vi "test TCX read (installed 71).vi"() -> ()   [LabVIEW 2011] (continued)
50</Watts></TPX></Extensions></Trackpoint><Trackpoint><Time>2008-03-03T13:52:56Z</Time><Position><LatitudeDegrees>35.876040</LatitudeDegrees><LongitudeDegrees>-78.942872</LongitudeDegrees></Position><AltitudeMeters>71.755</AltitudeMeters><DistanceMeters>2722.578</DistanceMeters><Cadence>80</Cadence><Extensions><TPX xmlns=\"http://www.garmin.com/xmlschemas/ActivityExtension/v2\"><Watts>198</Watts></TPX></Extensions></Trackpoint><Trackpoint><Time>2008-03-03T13:52:57Z</Time><Position><LatitudeDegrees>35.876036</LatitudeDegrees><LongitudeDegrees>-78.942746</LongitudeDegrees></Position><AltitudeMeters>71.755</AltitudeMeters><DistanceMeters>2733.887</DistanceMeters><Cadence>79</Cadence><Extensions><TPX xmlns=\"http://www.garmin.com/xmlschemas/ActivityExtension/v2\"><Watts>206</Watts></TPX></Extensions></Trackpoint><Trackpoint><Time>2008-03-03T13:52:58Z</Time><Position><LatitudeDegrees>35.876038</LatitudeDegrees><LongitudeDegrees>-78.942624</LongitudeDegrees></Position><AltitudeMeters>71.755</AltitudeMeters><DistanceMeters>2744.982</DistanceMeters><Cadence>76</Cadence><Extensions><TPX xmlns=\"http://www.garmin.com/xmlschemas/ActivityExtension/v2\"><Watts>226</Watts></TPX></Extensions></Trackpoint><Trackpoint><Time>2008-03-03T13:52:59Z</Time><Position><LatitudeDegrees>35.876041</LatitudeDegrees><LongitudeDegrees>-78.942503</LongitudeDegrees></Position><AltitudeMeters>72.236</AltitudeMeters><DistanceMeters>2755.792</DistanceMeters><Cadence>76</Cadence><Extensions><TPX xmlns=\"http://www.garmin.com/xmlschemas/ActivityExtension/v2\"><Watts>230</Watts></TPX></Extensions></Trackpoint><Trackpoint><Time>2008-03-03T13:53:00Z</Time><Position><LatitudeDegrees>35.876046</LatitudeDegrees><LongitudeDegrees>-78.942386</LongitudeDegrees></Position><AltitudeMeters>71.755</AltitudeMeters><DistanceMeters>2766.434</DistanceMeters><Cadence>76</Cadence><Extensions><TPX xmlns=\"http://www.garmin.com/xmlschemas/ActivityExtension/v2\"><Watts>228</Watts></TPX></Extensions></Trackpoint><Trackpoint><Time>2008-03-03T13:53:01Z</Time><Position><LatitudeDegrees>35.876052</LatitudeDegrees><LongitudeDegrees>-78.942271</LongitudeDegrees></Position><AltitudeMeters>72.236</AltitudeMeters><DistanceMeters>2776.748</DistanceMeters><Cadence>73</Cadence><Extensions><TPX xmlns=\"http://www.garmin.com/xmlschemas/ActivityExtension/v2\"><Watts>231</Watts></TPX></Extensions></Trackpoint><Trackpoint><Time>2008-03-03T13:53:02Z</Time><Position><LatitudeDegrees>35.876061</LatitudeDegrees><LongitudeDegrees>-78.942160</LongitudeDegrees></Position><AltitudeMeters>72.236</AltitudeMeters><DistanceMeters>2786.833</DistanceMeters><Cadence>71</Cadence><Extensions><TPX xmlns=\"http://www.garmin.com/xmlschemas/ActivityExtension/v2\"><Watts>227</Watts></TPX></Extensions></Trackpoint><Trackpoint><Time>2008-03-03T13:53:03Z</Time><Position><LatitudeDegrees>35.876074</LatitudeDegrees><LongitudeDegrees>-78.942052</LongitudeDegrees></Position><AltitudeMeters>72.236</AltitudeMeters><DistanceMeters>2796.726</DistanceMeters><Cadence>68</Cadence><Extensions><TPX xmlns=\"http://www.garmin.com/xmlschemas/ActivityExtension/v2\"><Watts>222</Watts></TPX></Extensions></Trackpoint><Trackpoint><Time>2008-03-03T13:53:04Z</Time><Position><LatitudeDegrees>35.876089</LatitudeDegrees><LongitudeDegrees>-78.941947</LongitudeDegrees></Position><AltitudeMeters>72.717</AltitudeMeters><DistanceMeters>2806.305</DistanceMeters><Cadence>68</Cadence><Extensions><TPX xmlns=\"http://www.garmin.com/xmlschemas/ActivityExtension/v2\"><Watts>231</Watts></TPX></Extensions></Trackpoint><Trackpoint><Time>2008-03-03T13:53:05Z</Time><Position><LatitudeDegrees>35.876106</LatitudeDegrees><LongitudeDegrees>-78.941844</LongitudeDegrees></Position><AltitudeMeters>72.717</AltitudeMeters><DistanceMeters>2815.787</DistanceMeters><Cadence>68</Cadence><Extensions><TPX xmlns=\"http://www.garmin.com/xmlschemas/ActivityExtension/v2\"><Watts>230</Watts></TPX></Extensions></Trackpoint><Trackpoint><Time>2008-03-03T13:53:06Z</Time><Position><LatitudeDegrees>35.876126</LatitudeDegrees><LongitudeDegrees>-78.941745</LongitudeDegrees></Position><AltitudeMeters>72.717</AltitudeMeters><DistanceMeters>2824.935</DistanceMeters><Cadence>65</Cadence><Extensions><TPX xmlns=\"http://www.garmin.com/xmlschemas/ActivityExtension/v2\"><Watts>244</Watts></TPX></Extensions></Trackpoint><Trackpoint><Time>2008-03-03T13:53:07Z</Time><Position><LatitudeDegrees>35.876144</LatitudeDegrees><LongitudeDegrees>-78.941647</LongitudeDegrees></Position><AltitudeMeters>73.198</AltitudeMeters><DistanceMeters>2834.040</DistanceMeters><Cadence>63</Cadence><Extensions><TPX xmlns=\"http://www.garmin.com/xmlschemas/ActivityExtension/v2\"><Watts>230</Watts></TPX></Extensions></Trackpoint><Trackpoint><Time>2008-03-03T13:53:08Z</Time><Position><LatitudeDegrees>35.876160</LatitudeDegrees><LongitudeDegrees>-78.941550</LongitudeDegrees></Position><AltitudeMeters>73.198</AltitudeMeters><DistanceMeters>2842.936</DistanceMeters><Cadence>62</Cadence><Extensions><TPX xmlns=\"http://www.garmin.com/xmlschemas/ActivityExtension/v2\"><Watts>222</Watts></TPX></Extensions></Trackpoint><Trackpoint><Time>2008-03-03T13:53:09Z</Time><Position><LatitudeDegrees>35.876180</LatitudeDegrees><LongitudeDegrees>-78.941457</LongitudeDegrees></Position><AltitudeMeters>73.678</AltitudeMeters><DistanceMeters>2851.633</DistanceMeters><Cadence>62</Cadence><Extensions><TPX xmlns=\"http://www.garmin.com/xmlschemas/ActivityExtension/v2\"><Watts>213</Watts></TPX></Extensions></Trackpoint><Trackpoint><Time>2008-03-03T13:53:10Z</Time><Position><LatitudeDegrees>35.876199</LatitudeDegrees><LongitudeDegrees>-78.941364</LongitudeDegrees></Position><AltitudeMeters>73.678</AltitudeMeters><DistanceMeters>2860.265</DistanceMeters><Cadence>66</Cadence><Extensions><TPX xmlns=\"http://www.garmin.com/xmlschemas/ActivityExtension/v2\"><Watts>203</Watts></TPX></Extensions></Trackpoint><Trackpoint><Time>2008-03-03T13:53:11Z</Time><Position><LatitudeDegrees>35.876216</LatitudeDegrees><LongitudeDegrees>-78.941272</LongitudeDegrees></Position><AltitudeMeters>73.678</AltitudeMeters><DistanceMeters>2868.794</DistanceMeters><Cadence>68</Cadence><Extensions><TPX xmlns=\"http://www.garmin.com/xmlschemas/ActivityExtension/v2\"><Watts>194</Watts></TPX></Extensions></Trackpoint><Trackpoint><Time>2008-03-03T13:53:12Z</Time><Position><LatitudeDegrees>35.876234</LatitudeDegrees><LongitudeDegrees>-78.941181</LongitudeDegrees></Position><AltitudeMeters>74.159</AltitudeMeters><DistanceMeters>2877.271</DistanceMeters><Cadence>69</Cadence><Extensions><TPX xmlns=\"http://www.garmin.com/xmlschemas/ActivityExtension/v2\"><Watts>188</Watts></TPX></Extensions></Trackpoint><Trackpoint><Time>2008-03-03T13:53:13Z</Time><Position><LatitudeDegrees>35.876255</LatitudeDegrees><LongitudeDegrees>-78.941091</LongitudeDegrees></Position><AltitudeMeters>73.198</AltitudeMeters><DistanceMeters>2885.719</DistanceMeters><Cadence>77</Cadence><Extensions><TPX xmlns=\"http://www.garmin.com/xmlschemas/ActivityExtension/v2\"><Watts>184</Watts></TPX></Extensions></Trackpoint><Trackpoint><Time>2008-03-03T13:53:14Z</Time><Position><LatitudeDegrees>35.876274</LatitudeDegrees><LongitudeDegrees>-78.941001</LongitudeDegrees></Position><AltitudeMeters>73.678</AltitudeMeters><DistanceMeters>2894.048</DistanceMeters><Cadence>77</Cadence><Extensions><TPX xmlns=\"http://www.garmin.com/xmlschemas/ActivityExtension/v2\"><Watts>183</Watts></TPX></Extensions></Trackpoint><Trackpoint><Time>2008-03-03T13:53:15Z</Time><Position><LatitudeDegrees>35.876290</LatitudeDegrees><LongitudeDegrees>-78.940913</LongitudeDegrees></Position><AltitudeMeters>74.159</AltitudeMeters><DistanceMeters>2902.261</DistanceMeters><Cadence>76</Cadence><Extensions><TPX xmlns=\"http://www.garmin.com/xmlschemas/ActivityExtension/v2\"><Watts>198</Watts></TPX></Extensions></Trackpoint><Trackpoint><Time>2008-03-03T13:53:16Z</Time><Position><LatitudeDegrees>35.876307</LatitudeDegrees><LongitudeDegrees>-78.940824</LongitudeDegrees></Position><AltitudeMeters>73.678</AltitudeMeters><DistanceMeters>2910.497</DistanceMeters><Cadence>76</Cadence><Extensions><TPX xmlns=\"http://www.garmin.com/xmlschemas/ActivityExtension/v2\"><Watts>206</Watts></TPX></Extensions></Trackpoint><Trackpoint><Time>2008-03-03T13:53:17Z</Time><Position><LatitudeDegrees>35.876319</LatitudeDegrees><LongitudeDegrees>-78.940734</LongitudeDegrees></Position><AltitudeMeters>74.159</AltitudeMeters><DistanceMeters>2918.685</DistanceMeters><Cadence>76</Cadence><Extensions><TPX xmlns=\"http://www.garmin.com/xmlschemas/ActivityExtension/v2\"><Watts>206</Watts></TPX></Extensions></Trackpoint><Trackpoint><Time>2008-03-03T13:53:18Z</Time><Position><LatitudeDegrees>35.876326</LatitudeDegrees><LongitudeDegrees>-78.940644</LongitudeDegrees></Position><AltitudeMeters>74.159</AltitudeMeters><DistanceMeters>2926.918</DistanceMeters><Cadence>76</Cadence><Extensions><TPX xmlns=\"http://www.garmin.com/xmlschemas/ActivityExtension/v2\"><Watts>198</Watts></TPX></Extensions></Trackpoint><Trackpoint><Time>2008-03-03T13:53:19Z</Time><Position><LatitudeDegrees>35.876330</LatitudeDegrees><LongitudeDegrees>-78.940552</LongitudeDegrees></Position><AltitudeMeters>73.678</AltitudeMeters><DistanceMeters>2935.164</DistanceMeters><Cadence>77</Cadence><Extensions><TPX xmlns=\"http://www.garmin.com/xmlschemas/ActivityExtension/v2\"><Watts>178</Watts></TPX></Extensions></Trackpoint><Trackpoint><Time>2008-03-03T13:53:20Z</Time><Position><LatitudeDegrees>35.876336</LatitudeDegrees><LongitudeDegrees>-78.940461</LongitudeDegrees></Position><AltitudeMeters>73.678</AltitudeMeters><DistanceMeters>2943.486</DistanceMeters><Cadence>77</Cadence><Extensions><TPX xmlns=\"http://www.garmin.com/xmlschemas/ActivityExtension/v2\"><Watts>165</Watts></TPX></Extensions></Trackpoint><Trackpoint><Time>2008-03-03T13:53:21Z</Time><Position><LatitudeDegrees>35.876341</LatitudeDegrees><LongitudeDegrees>-78.940369</LongitudeDegrees></Position><AltitudeMeters>74.640</AltitudeMeters><DistanceMeters>2951.737</DistanceMeters><Cadence>78</Cadence><Extensions><TPX xmlns=\"http://www.garmin.com/xmlschemas/ActivityExtension/v2\"><Watts>167</Watts></TPX></Extensions></Trackpoint><Trackpoint><Time>2008-03-03T13:53:22Z</Time><Position><LatitudeDegrees>35.876344</LatitudeDegrees><LongitudeDegrees>-78.940279</LongitudeDegrees></Position><AltitudeMeters>74.159</AltitudeMeters><DistanceMeters>2959.913</DistanceMeters><Cadence>77</Cadence><Extensions><TPX xmlns=\"http://www.garmin.com/xmlschemas/ActivityExtension/v2\"><Watts>184</Watts></TPX></Extensions></Trackpoint><Trackpoint><Time>2008-03-03T13:53:23Z</Time><Position><LatitudeDegrees>35.876339</LatitudeDegrees><LongitudeDegrees>-78.940189</LongitudeDegrees></Position><AltitudeMeters>74.159</AltitudeMeters><DistanceMeters>2968.036</DistanceMeters><Cadence>75</Cadence><Extensions><TPX xmlns=\"http://www.garmin.com/xmlschemas/ActivityExtension/v2\"><Watts>193</Watts></TPX></Extensions></Trackpoint><Trackpoint><Time>2008-03-03T13:53:24Z</Time><Position><LatitudeDegrees>35.876329</LatitudeDegrees><LongitudeDegrees>-78.940101</LongitudeDegrees></Position><AltitudeMeters>74.640</AltitudeMeters><DistanceMeters>2976.068</DistanceMeters><Cadence>75</Cadence><Extensions><TPX xmlns=\"http://www.garmin.com/xmlschemas/ActivityExtension/v2\"><Watts>188</Watts></TPX></Extensions></Trackpoint><Trackpoint><Time>2008-03-03T13:53:25Z</Time><Position><LatitudeDegrees>35.876319</LatitudeDegrees><LongitudeDegrees>-78.940014</LongitudeDegrees></Position><AltitudeMeters>74.159</AltitudeMeters><DistanceMeters>2983.947</DistanceMeters><Cadence>73</Cadence><Extensions><TPX xmlns=\"http://www.garmin.com/xmlschemas/ActivityExtension/v2\"><Watts>181</Watts></TPX></Extensions></Trackpoint><Trackpoint><Time>2008-03-03T13:53:26Z</Time><Position><LatitudeDegrees>35.876312</LatitudeDegrees><LongitudeDegrees>-78.939931</LongitudeDegrees></Position><AltitudeMeters>75.120</AltitudeMeters><DistanceMeters>2991.509</DistanceMeters><Cadence>72</Cadence><Extensions><TPX xmlns=\"http://www.garmin.com/xmlschemas/ActivityExtension/v2\"><Watts>188</Watts></TPX></Extensions></Trackpoint><Trackpoint><Time>2008-03-03T13:53:27Z</Time><Position><LatitudeDegrees>35.876298</LatitudeDegrees><LongitudeDegrees>-78.939849</LongitudeDegrees></Position><AltitudeMeters>75.120</AltitudeMeters><DistanceMeters>2999.027</DistanceMeters><Cadence>70</Cadence><Extensions><TPX xmlns=\"http://www.garmin.com/xmlschemas/ActivityExtension/v2\"><Watts>193</Watts></TPX></Extensions></Trackpoint><Trackpoint><Time>2008-03-03T13:53:28Z</Time><Position><LatitudeDegrees>35.876283</LatitudeDegrees><LongitudeDegrees>-78.939770</LongitudeDegrees></Position><AltitudeMeters>75.120</AltitudeMeters><DistanceMeters>3006.346</DistanceMeters><Cadence>68</Cadence><Extensions><TPX xmlns=\"http://www.garmin.com/xmlschemas/ActivityExtension/v2\"><Watts>212</Watts></TPX></Extensions></Trackpoint><Trackpoint><Time>2008-03-03T13:53:29Z</Time><Position><LatitudeDegrees>35.876270</LatitudeDegrees><LongitudeDegrees>-78.939695</LongitudeDegrees></Position><AltitudeMeters>75.120</AltitudeMeters><DistanceMeters>3013.253</DistanceMeters><Cadence>66</Cadence><Extensions><TPX xmlns=\"http://www.garmin.com/xmlschemas/ActivityExtension/v2\"><Watts>213</Watts></TPX></Extensions></Trackpoint><Trackpoint><Time>2008-03-03T13:53:30Z</Time><Position><LatitudeDegrees>35.876249</LatitudeDegrees><LongitudeDegrees>-78.939622</LongitudeDegrees></Position><AltitudeMeters>75.601</AltitudeMeters><DistanceMeters>3020.261</DistanceMeters><Cadence>69</Cadence><Extensions><TPX xmlns=\"http://www.garmin.com/xmlschemas/ActivityExtension/v2\"><Watts>207</Watts></TPX></Extensions></Trackpoint><Trackpoint><Time>2008-03-03T13:53:31Z</Time><Position><LatitudeDegrees>35.876226</LatitudeDegrees><LongitudeDegrees>-78.939552</LongitudeDegrees></Position><AltitudeMeters>75.601</AltitudeMeters><DistanceMeters>3027.026</DistanceMeters><Cadence>70</Cadence><Extensions><TPX xmlns=\"http://www.garmin.com/xmlschemas/ActivityExtension/v2\"><Watts>190</Watts></TPX></Extensions></Trackpoint><Trackpoint><Time>2008-03-03T13:53:32Z</Time><Position><LatitudeDegrees>35.876204</LatitudeDegrees><LongitudeDegrees>-78.939484</LongitudeDegrees></Position><AltitudeMeters>76.081</AltitudeMeters><DistanceMeters>3033.609</DistanceMeters><Cadence>70</Cadence><Extensions><TPX xmlns=\"http://www.garmin.com/xmlschemas/ActivityExtension/v2\"><Watts>190</Watts></TPX></Extensions></Trackpoint><Trackpoint><Time>2008-03-03T13:53:33Z</Time><Position><LatitudeDegrees>35.876179</LatitudeDegrees><LongitudeDegrees>-78.939418</LongitudeDegrees></Position><AltitudeMeters>76.081</AltitudeMeters><DistanceMeters>3040.216</DistanceMeters><Cadence>67</Cadence><Extensions><TPX xmlns=\"http://www.garmin.com/xmlschemas/ActivityExtension/v2\"><Watts>190</Watts></TPX></Extensions></Trackpoint><Trackpoint><Time>2008-03-03T13:53:34Z</Time><Position><LatitudeDegrees>35.876153</LatitudeDegrees><LongitudeDegrees>-78.939354</LongitudeDegrees></Position><AltitudeMeters>76.562</AltitudeMeters><DistanceMeters>3046.654</DistanceMeters><Cadence>66</Cadence><Extensions><TPX xmlns=\"http://www.garmin.com/xmlschemas/ActivityExtension/v2\"><Watts>212</Watts></TPX></Extensions></Trackpoint><Trackpoint><Time>2008-03-03T13:53:35Z</Time><Position><LatitudeDegrees>35.876126</LatitudeDegrees><LongitudeDegrees>-78.939291</LongitudeDegrees></Position><AltitudeMeters>76.562</AltitudeMeters><DistanceMeters>3053.088</DistanceMeters><Cadence>66</Cadence><Extensions><TPX xmlns=\"http://www.garmin.com/xmlschemas/ActivityExtension/v2\"><Watts>221</Watts></TPX></Extensions></Trackpoint><Trackpoint><Time>2008-03-03T13:53:36Z</Time><Position><LatitudeDegrees>35.876095</LatitudeDegrees><LongitudeDegrees>-78.939230</LongitudeDegrees></Position><AltitudeMeters>76.562</AltitudeMeters><DistanceMeters>3059.617</DistanceMeters><Cadence>65</Cadence><Extensions><TPX xmlns=\"http://www.garmin.com/xmlschemas/ActivityExtension/v2\"><Watts>223</Watts></TPX></Extensions></Trackpoint><Trackpoint><Time>2008-03-03T13:53:37Z</Time><Position><LatitudeDegrees>35.876065</LatitudeDegrees><LongitudeDegrees>-78.939170</LongitudeDegrees></Position><AltitudeMeters>77.043</AltitudeMeters><DistanceMeters>3065.932</DistanceMeters><Cadence>65</Cadence><Extensions><TPX xmlns=\"http://www.garmin.com/xmlschemas/ActivityExtension/v2\"><Watts>224</Watts></TPX></Extensions></Trackpoint><Trackpoint><Time>2008-03-03T13:53:38Z</Time><Position><LatitudeDegrees>35.876040</LatitudeDegrees><LongitudeDegrees>-78.939114</LongitudeDegrees></Position><AltitudeMeters>77.523</AltitudeMeters><DistanceMeters>3071.715</DistanceMeters><Cadence>65</Cadence><Extensions><TPX xmlns=\"http://www.garmin.com/xmlschemas/ActivityExtension/v2\"><Watts>285</Watts></TPX></Extensions></Trackpoint><Trackpoint><Time>2008-03-03T13:53:39Z</Time><Position><LatitudeDegrees>35.876013</LatitudeDegrees><LongitudeDegrees>-78.939058</LongitudeDegrees></Position><AltitudeMeters>77.523</AltitudeMeters><DistanceMeters>3077.505</DistanceMeters><Cadence>65</Cadence><Extensions><TPX xmlns=\"http://www.garmin.com/xmlschemas/ActivityExtension/v2\"><Watts>287</Watts></TPX></Extensions></Trackpoint><Trackpoint><Time>2008-03-03T13:53:40Z</Time><Position><LatitudeDegrees>35.875986</LatitudeDegrees><LongitudeDegrees>-78.939004</LongitudeDegrees></Position><AltitudeMeters>77.523</AltitudeMeters><DistanceMeters>3083.213</DistanceMeters><Cadence>62</Cadence><Extensions><TPX xmlns=\"http://www.garmin.com/xmlschemas/ActivityExtension/v2\"><Watts>298</Watts></TPX></Extensions></Trackpoint><Trackpoint><Time>2008-03-03T13:53:41Z</Time><Position><LatitudeDegrees>35.875957</LatitudeDegrees><LongitudeDegrees>-78.938951</LongitudeDegrees></Position><AltitudeMeters>78.004</AltitudeMeters><DistanceMeters>3088.980</DistanceMeters><Cadence>59</Cadence><Extensions><TPX xmlns=\"http://www.garmin.com/xmlschemas/ActivityExtension/v2\"><Watts>286</Watts></TPX></Extensions></Trackpoint><Trackpoint><Time>2008-03-03T13:53:42Z</Time><Position><LatitudeDegrees>35.875930</LatitudeDegrees><LongitudeDegrees>-78.938899</LongitudeDegrees></Position><AltitudeMeters>78.485</AltitudeMeters><DistanceMeters>3094.533</DistanceMeters><Cadence>59</Cadence><Extensions><TPX xmlns=\"http://www.garmin.com/xmlschemas/ActivityExtension/v2\"><Watts>266</Watts></TPX></Extensions></Trackpoint><Trackpoint><Time>2008-03-03T13:53:43Z</Time><Position><LatitudeDegrees>35.875901</LatitudeDegrees><LongitudeDegrees>-78.938849</LongitudeDegrees></Position><AltitudeMeters>78.965</AltitudeMeters><DistanceMeters>3100.031</DistanceMeters><Cadence>64</Cadence><Extensions><TPX xmlns=\"http://www.garmin.com/xmlschemas/ActivityExtension/v2\"><Watts>273</Watts></TPX></Extensions></Trackpoint><Trackpoint><Time>2008-03-03T13:53:44Z</Time><Position><LatitudeDegrees>35.875879</LatitudeDegrees><LongitudeDegrees>-78.938802</LongitudeDegrees></Position><AltitudeMeters>78.965</AltitudeMeters><DistanceMeters>3104.980</DistanceMeters><Cadence>64</Cadence><Extensions><TPX xmlns=\"http://www.garmin.com/xmlschemas/ActivityExtension/v2\"><Watts>272</Watts></TPX></Extensions></Trackpoint><Trackpoint><Time>2008-03-03T13:53:45Z</Time><Position><LatitudeDegrees>35.875860</LatitudeDegrees><LongitudeDegrees>-78.938755</LongitudeDegrees></Position><AltitudeMeters>79.446</AltitudeMeters><DistanceMeters>3109.719</DistanceMeters><Cadence>63</Cadence><Extensions><TPX xmlns=\"http://www.garmin.com/xmlschemas/ActivityExtension/v2\"><Watts>321</Watts></TPX></Extensions></Trackpoint><Trackpoint><Time>2008-03-03T13:53:46Z</Time><Position><LatitudeDegrees>35.875841</LatitudeDegrees><LongitudeDegrees>-78.938706</LongitudeDegrees></Position><AltitudeMeters>79.927</AltitudeMeters><DistanceMeters>3114.581</DistanceMeters><Cadence>66</Cadence><Extensions><TPX xmlns=\"http://www.garmin.com/xmlschemas/ActivityExtension/v2\"><Watts>408</Watts></TPX></Extensions></Trackpoint><Trackpoint><Time>2008-03-03T13:53:47Z</Time><Position><LatitudeDegrees>35.875815</LatitudeDegrees><LongitudeDegrees>-78.938655</LongitudeDegrees></Position><AltitudeMeters>80.888</AltitudeMeters><DistanceMeters>3120.059</DistanceMeters><Cadence>67</Cadence><Extensions><TPX xmlns=\"http://www.garmin.com/xmlschemas/ActivityExtension/v2\"><Watts>494</Watts></TPX></Extensions></Trackpoint><Trackpoint><Time>2008-03-03T13:53:48Z</Time><Position><LatitudeDegrees>35.875794</LatitudeDegrees><LongitudeDegrees>-78.938603</LongitudeDegrees></Position><AltitudeMeters>80.888</AltitudeMeters><DistanceMeters>3125.269</DistanceMeters><Cadence>69</Cadence><Extensions><TPX xmlns=\"http://www.garmin.com/xmlschemas/ActivityExtension/v2\"><Watts>550</Watts></TPX></Extensions></Trackpoint><Trackpoint><Time>2008-03-03T13:53:49Z</Time><Position><LatitudeDegrees>35.875770</LatitudeDegrees><LongitudeDegrees>-78.938550</LongitudeDegrees></Position><AltitudeMeters>81.369</AltitudeMeters><DistanceMeters>3130.710</DistanceMeters><Cadence>69</Cadence><Extensions><TPX xmlns=\"http://www.garmin.com/xmlschemas/ActivityExtension/v2\"><Watts>568</Watts></TPX></Extensions></Trackpoint><Trackpoint><Time>2008-03-03T13:53:50Z</Time><Position><LatitudeDegrees>35.875740</LatitudeDegrees><LongitudeDegrees>-78.938499</LongitudeDegrees></Position><AltitudeMeters>82.330</AltitudeMeters><DistanceMeters>3136.402</DistanceMeters><Cadence>71</Cadence><Extensions><TPX xmlns=\"http://www.garmin.com/xmlschemas/ActivityExtension/v2\"><Watts>622</Watts></TPX></Extensions></Trackpoint><Trackpoint><Time>2008-03-03T13:53:51Z</Time><Position><LatitudeDegrees>35.875712</LatitudeDegrees><LongitudeDegrees>-78.938449</LongitudeDegrees></Position><AltitudeMeters>82.330</AltitudeMeters><DistanceMeters>3141.893</DistanceMeters><Cadence>71</Cadence><Extensions><TPX xmlns=\"http://www.garmin.com/xmlschemas/ActivityExtension/v2\"><Watts>621</Watts></TPX></Extensions></Trackpoint><Trackpoint><Time>2008-03-03T13:53:52Z</Time><Position><LatitudeDegrees>35.875682</LatitudeDegrees><LongitudeDegrees>-78.938393</LongitudeDegrees></Position><AltitudeMeters>83.291</AltitudeMeters><DistanceMeters>3147.943</DistanceMeters><Cadence>73</Cadence><Extensions><TPX xmlns=\"http://www.garmin.com/xmlschemas/ActivityExtension/v2\"><Watts>636</Watts></TPX></Extensions></Trackpoint><Trackpoint><Time>2008-03-03T13:53:53Z</Time><Position><LatitudeDegrees>35.875648</LatitudeDegrees><LongitudeDegrees>-78.938334</LongitudeDegrees></Position><AltitudeMeters>83.772</AltitudeMeters><DistanceMeters>3154.416</DistanceMeters><Cadence>75</Cadence><Extensions><TPX xmlns=\"http://www.garmin.com/xmlschemas/ActivityExtension/v2\"><Watts>637</Watts></TPX></Extensions></Trackpoint><Trackpoint><Time>2008-03-03T13:53:54Z</Time><Position><LatitudeDegrees>35.875619</LatitudeDegrees><LongitudeDegrees>-78.938279</LongitudeDegrees></Position><AltitudeMeters>84.253</AltitudeMeters><DistanceMeters>3160.336</DistanceMeters><Cadence>76</Cadence><Extensions><TPX xmlns=\"http://www.garmin.com/xmlschemas/ActivityExtension/v2\"><Watts>637</Watts></TPX></Extensions></Trackpoint><Trackpoint><Time>2008-03-03T13:53:55Z</Time><Position><LatitudeDegrees>35.875599</LatitudeDegrees><LongitudeDegrees>-78.938225</LongitudeDegrees></Position><AltitudeMeters>84.733</AltitudeMeters><DistanceMeters>3165.657</DistanceMeters><Cadence>76</Cadence><Extensions><TPX xmlns=\"http://www.garmin.com/xmlschemas/ActivityExtension/v2\"><Watts>646</Watts></TPX></Extensions></Trackpoint><Trackpoint><Time>2008-03-03T13:53:56Z</Time><Position><LatitudeDegrees>35.875579</LatitudeDegrees><LongitudeDegrees>-78.938169</LongitudeDegrees></Position><AltitudeMeters>85.695</AltitudeMeters><DistanceMeters>3171.157</DistanceMeters><Cadence>76</Cadence><Extensions><TPX xmlns=\"http://www.garmin.com/xmlschemas/ActivityExtension/v2\"><Watts>648</Watts></TPX></Extensions></Trackpoint><Trackpoint><Time>2008-03-03T13:53:57Z</Time><Position><LatitudeDegrees>35.875551</LatitudeDegrees><LongitudeDegrees>-78.938110</LongitudeDegrees></Position><AltitudeMeters>86.175</AltitudeMeters><DistanceMeters>3177.342</DistanceMeters><Cadence>76</Cadence><Extensions><TPX xmlns=\"http://www.garmin.com/xmlschemas/ActivityExtension/v2\"><Watts>649</Watts></TPX></Extensions></Trackpoint><Trackpoint><Time>2008-03-03T13:53:58Z</Time><Position><LatitudeDegrees>35.875518</LatitudeDegrees><LongitudeDegrees>-78.938054</LongitudeDegrees></Position><AltitudeMeters>86.656</AltitudeMeters><DistanceMeters>3183.580</DistanceMeters><Cadence>75</Cadence><Extensions><TPX xmlns=\"http://www.garmin.com/xmlschemas/ActivityExtension/v2\"><Watts>631</Watts></TPX></Extensions></Trackpoint><Trackpoint><Time>2008-03-03T13:53:59Z</Time><Position><LatitudeDegrees>35.875485</LatitudeDegrees><LongitudeDegrees>-78.937997</LongitudeDegrees></Position><AltitudeMeters>87.137</AltitudeMeters><DistanceMeters>3189.851</DistanceMeters><Cadence>75</Cadence><Extensions><TPX xmlns=\"http://www.garmin.com/xmlschemas/ActivityExtension/v2\"><Watts>638</Watts></TPX></Extensions></Trackpoint><Trackpoint><Time>2008-03-03T13:54:00Z</Time><Position><LatitudeDegrees>35.875451</LatitudeDegrees><LongitudeDegrees>-78.937941</LongitudeDegrees></Position><AltitudeMeters>87.617</AltitudeMeters><DistanceMeters>3196.059</DistanceMeters><Cadence>72</Cadence><Extensions><TPX xmlns=\"http://www.garmin.com/xmlschemas/ActivityExtension/v2\"><Watts>598</Watts></TPX></Extensions></Trackpoint><Trackpoint><Time>2008-03-03T13:54:01Z</Time><Position><LatitudeDegrees>35.875417</LatitudeDegrees><LongitudeDegrees>-78.937886</LongitudeDegrees></Position><AltitudeMeters>88.579</AltitudeMeters><DistanceMeters>3202.354</DistanceMeters><Cadence>72</Cadence><Extensions><TPX xmlns=\"http://www.garmin.com/xmlschemas/ActivityExtension/v2\"><Watts>598</Watts></TPX></Extensions></Trackpoint><Trackpoint><Time>2008-03-03T13:54:02Z</Time><Position><LatitudeDegrees>35.875381</LatitudeDegrees><LongitudeDegrees>-78.937831</LongitudeDegrees></Position><AltitudeMeters>89.059</AltitudeMeters><DistanceMeters>3208.651</DistanceMeters><Cadence>72</Cadence><Extensions><TPX xmlns=\"http://www.garmin.com/xmlschemas/ActivityExtension/v2\"><Watts>579</Watts></TPX></Extensions></Trackpoint><Trackpoint><Time>2008-03-03T13:54:03Z</Time><Position><LatitudeDegrees>35.875355</LatitudeDegrees><LongitudeDegrees>-78.937771</LongitudeDegrees></Position><AltitudeMeters>89.540</AltitudeMeters><DistanceMeters>3214.748</DistanceMeters><Cadence>72</Cadence><Extensions><TPX xmlns=\"http://www.garmin.com/xmlschemas/ActivityExtension/v2\"><Watts>560</Watts></TPX></Extensions></Trackpoint><Trackpoint><Time>2008-03-03T13:54:04Z</Time><Position><LatitudeDegrees>35.875324</LatitudeDegrees><LongitudeDegrees>-78.937713</LongitudeDegrees></Position><AltitudeMeters>90.021</AltitudeMeters><DistanceMeters>3220.997</DistanceMeters><Cadence>72</Cadence><Extensions><TPX xmlns=\"http://www.garmin.com/xmlschemas/ActivityExtension/v2\"><Watts>561</Watts></TPX></Extensions></Trackpoint><Trackpoint><Time>2008-03-03T13:54:05Z</Time><Position><LatitudeDegrees>35.875292</LatitudeDegrees><LongitudeDegrees>-78.937656</LongitudeDegrees></Position><AltitudeMeters>90.501</AltitudeMeters><DistanceMeters>3227.245</DistanceMeters><Cadence>73</Cadence><Extensions><TPX xmlns=\"http://www.garmin.com/xmlschemas/ActivityExtension/v2\"><Watts>559</Watts></TPX></Extensions></Trackpoint><Trackpoint><Time>2008-03-03T13:54:06Z</Time><Position><LatitudeDegrees>35.875264</LatitudeDegrees><LongitudeDegrees>-78.937595</LongitudeDegrees></Position><AltitudeMeters>90.501</AltitudeMeters><DistanceMeters>3233.512</DistanceMeters><Cadence>72</Cadence><Extensions><TPX xmlns=\"http://www.garmin.com/xmlschemas/ActivityExtension/v2\"><Watts>546</Watts></TPX></Extensions></Trackpoint><Trackpoint><Time>2008-03-03T13:54:07Z</Time><Position><LatitudeDegrees>35.875235</LatitudeDegrees><LongitudeDegrees>-78.937534</LongitudeDegrees></Position><AltitudeMeters>90.982</AltitudeMeters><DistanceMeters>3239.940</DistanceMeters><Cadence>74</Cadence><Extensions><TPX xmlns=\"http://www.garmin.com/xmlschemas/ActivityExtension/v2\"><Watts>481</Watts></TPX></Extensions></Trackpoint><Trackpoint><Time>2008-03-03T13:54:08Z</Time><Position><LatitudeDegrees>35.875204</LatitudeDegrees><LongitudeDegrees>-78.937474</LongitudeDegrees></Position><AltitudeMeters>91.463</AltitudeMeters><DistanceMeters>3246.413</DistanceMeters><Cadence>77</Cadence><Extensions><TPX xmlns=\"http://www.garmin.com/xmlschemas/ActivityExtension/v2\"><Watts>448</Watts></TPX></Extensions></Trackpoint><Trackpoint><Time>2008-03-03T13:54:09Z</Time><Position><LatitudeDegrees>35.875176</LatitudeDegrees><LongitudeDegrees>-78.937420</LongitudeDegrees></Position><AltitudeMeters>91.943</AltitudeMeters><DistanceMeters>3252.062</DistanceMeters><Cadence>77</Cadence><Extensions><TPX xmlns=\"http://www.garmin.com/xmlschemas/ActivityExtension/v2\"><Watts>449</Watts></TPX></Extensions></Trackpoint><Trackpoint><Time>2008-03-03T13:54:10Z</Time><Position><LatitudeDegrees>35.875150</LatitudeDegrees><LongitudeDegrees>-78.937367</LongitudeDegrees></Position><AltitudeMeters>91.943</AltitudeMeters><DistanceMeters>3257.750</DistanceMeters><Cadence>70</Cadence><Extensions><TPX xmlns=\"http://www.garmin.com/xmlschemas/ActivityExtension/v2\"><Watts>302</Watts></TPX></Extensions></Trackpoint><Trackpoint><Time>2008-03-03T13:54:11Z</Time><Position><LatitudeDegrees>35.875123</LatitudeDegrees><LongitudeDegrees>-78.937309</LongitudeDegrees></Position><AltitudeMeters>91.943</AltitudeMeters><DistanceMeters>3263.753</DistanceMeters><Cadence>70</Cadence><Extensions><TPX xmlns=\"http://www.garmin.com/xmlschemas/ActivityExtension/v2\"><Watts>238</Watts></TPX></Extensions></Trackpoint><Trackpoint><Time>2008-03-03T13:54:12Z</Time><Position><LatitudeDegrees>35.875097</LatitudeDegrees><LongitudeDegrees>-78.937251</LongitudeDegrees></Position><AltitudeMeters>92.424</AltitudeMeters><DistanceMeters>3269.682</DistanceMeters><Cadence>69</Cadence><Extensions><TPX xmlns=\"http://www.garmin.com/xmlschemas/ActivityExtension/v2\"><Watts>223</Watts></TPX></Extensions></Trackpoint><Trackpoint><Time>2008-03-03T13:54:13Z</Time><Position><LatitudeDegrees>35.875074</LatitudeDegrees><LongitudeDegrees>-78.937193</LongitudeDegrees></Position><AltitudeMeters>92.424</AltitudeMeters><DistanceMeters>3275.529</DistanceMeters><Cadence>70</Cadence><Extensions><TPX xmlns=\"http://www.garmin.com/xmlschemas/ActivityExtension/v2\"><Watts>219</Watts></TPX></Extensions></Trackpoint><Trackpoint><Time>2008-03-03T13:54:14Z</Time><Position><LatitudeDegrees>35.875053</LatitudeDegrees><LongitudeDegrees>-78.937134</LongitudeDegrees></Position><AltitudeMeters>92.905</AltitudeMeters><DistanceMeters>3281.400</DistanceMeters><Cadence>70</Cadence><Extensions><TPX xmlns=\"http://www.garmin.com/xmlschemas/ActivityExtension/v2\"><Watts>217</Watts></TPX></Extensions></Trackpoint><Trackpoint><Time>2008-03-03T13:54:15Z</Time><Position><LatitudeDegrees>35.875031</LatitudeDegrees><LongitudeDegrees>-78.937073</LongitudeDegrees></Position><AltitudeMeters>92.424</AltitudeMeters><DistanceMeters>3287.417</DistanceMeters><Cadence>72</Cadence><Extensions><TPX xmlns=\"http://www.garmin.com/xmlschemas/ActivityExtension/v2\"><Watts>202</Watts></TPX></Extensions></Trackpoint><Trackpoint><Time>2008-03-03T13:54:16Z</Time><Position><LatitudeDegrees>35.875010</LatitudeDegrees><LongitudeDegrees>-78.937010</LongitudeDegrees></Position><AltitudeMeters>92.905</AltitudeMeters><DistanceMeters>3293.521</DistanceMeters><Cadence>72</Cadence><Extensions><TPX xmlns=\"http://www.garmin.com/xmlschemas/ActivityExtension/v2\"><Watts>202</Watts></TPX></Extensions></Trackpoint><Trackpoint><Time>2008-03-03T13:54:17Z</Time><Position><LatitudeDegrees>35.874991</LatitudeDegrees><LongitudeDegrees>-78.936946</LongitudeDegrees></Position><AltitudeMeters>92.905</AltitudeMeters><DistanceMeters>3299.711</DistanceMeters><Cadence>72</Cadence><Extensions><TPX xmlns=\"http://www.garmin.com/xmlschemas/ActivityExtension/v2\"><Watts>202</Watts></TPX></Extensions></Trackpoint><Trackpoint><Time>2008-03-03T13:54:18Z</Time><Position><LatitudeDegrees>35.874971</LatitudeDegrees><LongitudeDegrees>-78.936880</LongitudeDegrees></Position><AltitudeMeters>92.905</AltitudeMeters><DistanceMeters>3306.040</DistanceMeters><Cadence>74</Cadence><Extensions><TPX xmlns=\"http://www.garmin.com/xmlschemas/ActivityExtension/v2\"><Watts>202</Watts></TPX></Extensions></Trackpoint><Trackpoint><Time>2008-03-03T13:54:19Z</Time><Position><LatitudeDegrees>35.874958</LatitudeDegrees><LongitudeDegrees>-78.936815</LongitudeDegrees></Position><AltitudeMeters>92.905</AltitudeMeters><DistanceMeters>3312.117</DistanceMeters><Cadence>74</Cadence><Extensions><TPX xmlns=\"http://www.garmin.com/xmlschemas/ActivityExtension/v2\"><Watts>202</Watts></TPX></Extensions></Trackpoint><Trackpoint><Time>2008-03-03T13:54:20Z</Time><Position><LatitudeDegrees>35.874938</LatitudeDegrees><LongitudeDegrees>-78.936747</LongitudeDegrees></Position><AltitudeMeters>93.385</AltitudeMeters><DistanceMeters>3318.629</DistanceMeters><Cadence>74</Cadence><Extensions><TPX xmlns=\"http://www.garmin.com/xmlschemas/ActivityExtension/v2\"><Watts>200</Watts></TPX></Extensions></Trackpoint><Trackpoint><Time>2008-03-03T13:54:21Z</Time><Position><LatitudeDegrees>35.874921</LatitudeDegrees><LongitudeDegrees>-78.936679</LongitudeDegrees></Position><AltitudeMeters>93.385</AltitudeMeters><DistanceMeters>3325.057</DistanceMeters><Cadence>75</Cadence><Extensions><TPX xmlns=\"http://www.garmin.com/xmlschemas/ActivityExtension/v2\"><Watts>189</Watts></TPX></Extensions></Trackpoint><Trackpoint><Time>2008-03-03T13:54:22Z</Time><Position><LatitudeDegrees>35.874906</LatitudeDegrees><LongitudeDegrees>-78.936611</LongitudeDegrees></Position><AltitudeMeters>93.385</AltitudeMeters><DistanceMeters>3331.391</DistanceMeters><Cadence>74</Cadence><Extensions><TPX xmlns=\"http://www.garmin.com/xmlschemas/ActivityExtension/v2\"><Watts>164</Watts></TPX></Extensions></Trackpoint><Trackpoint><Time>2008-03-03T13:54:23Z</Time><Position><LatitudeDegrees>35.874892</LatitudeDegrees><LongitudeDegrees>-78.936543</LongitudeDegrees></Position><AltitudeMeters>93.385</AltitudeMeters><DistanceMeters>3337.708</DistanceMeters><Cadence>74</Cadence><Extensions><TPX xmlns=\"http://www.garmin.com/xmlschemas/ActivityExtension/v2\"><Watts>153</Watts></TPX></Extensions></Trackpoint><Trackpoint><Time>2008-03-03T13:54:24Z</Time><Position><LatitudeDegrees>35.874883</LatitudeDegrees><LongitudeDegrees>-78.936477</LongitudeDegrees></Position><AltitudeMeters>93.385</AltitudeMeters><DistanceMeters>3343.771</DistanceMeters><Cadence>73</Cadence><Extensions><TPX xmlns=\"http://www.garmin.com/xmlschemas/ActivityExtension/v2\"><Watts>145</Watts></TPX></Extensions></Trackpoint><Trackpoint><Time>2008-03-03T13:54:25Z</Time><Position><LatitudeDegrees>35.874874</LatitudeDegrees><LongitudeDegrees>-78.936409</LongitudeDegrees></Position><AltitudeMeters>93.385</AltitudeMeters><DistanceMeters>3349.997</DistanceMeters><Cadence>74</Cadence><Extensions><TPX xmlns=\"http://www.garmin.com/xmlschemas/ActivityExtension/v2\"><Watts>141</Watts></TPX></Extensions></Trackpoint><Trackpoint><Time>2008-03-03T13:54:26Z</Time><Position><LatitudeDegrees>35.874867</LatitudeDegrees><LongitudeDegrees>-78.936339</LongitudeDegrees></Position><AltitudeMeters>93.385</AltitudeMeters><DistanceMeters>3356.326</DistanceMeters><Cadence>74</Cadence><Extensions><TPX xmlns=\"http://www.garmin.com/xmlschemas/ActivityExtension/v2\"><Watts>139</Watts></TPX></Extensions></Trackpoint><Trackpoint><Time>2008-03-03T13:54:27Z</Time><Position><LatitudeDegrees>35.874858</LatitudeDegrees><LongitudeDegrees>-78.936269</LongitudeDegrees></Position><AltitudeMeters>93.866</AltitudeMeters><DistanceMeters>3362.754</DistanceMeters><Cadence>76</Cadence><Extensions><TPX xmlns=\"http://www.garmin.com/xmlschemas/ActivityExtension/v2\"><Watts>139</Watts></TPX></Extensions></Trackpoint><Trackpoint><Time>2008-03-03T13:54:28Z</Time><Position><LatitudeDegrees>35.874854</LatitudeDegrees><LongitudeDegrees>-78.936197</LongitudeDegrees></Position><AltitudeMeters>93.866</AltitudeMeters><DistanceMeters>3369.221</DistanceMeters><Cadence>76</Cadence><Extensions><TPX xmlns=\"http://www.garmin.com/xmlschemas/ActivityExtension/v2\"><Watts>138</Watts></TPX></Extensions></Trackpoint><Trackpoint><Time>2008-03-03T13:54:29Z</Time><Position><LatitudeDegrees>35.874852</LatitudeDegrees><LongitudeDegrees>-78.936125</LongitudeDegrees></Position><AltitudeMeters>93.866</AltitudeMeters><DistanceMeters>3375.744</DistanceMeters><Cadence>77</Cadence><Extensions><TPX xmlns=\"http://www.garmin.com/xmlschemas/ActivityExtension/v2\"><Watts>137</Watts></TPX></Extensions></Trackpoint><Trackpoint><Time>2008-03-03T13:54:30Z</Time><Position><LatitudeDegrees>35.874854</LatitudeDegrees><LongitudeDegrees>-78.936052</LongitudeDegrees></Position><AltitudeMeters>93.866</AltitudeMeters><DistanceMeters>3382.318</DistanceMeters><Cadence>79</Cadence><Extensions><TPX xmlns=\"http://www.garmin.com/xmlschemas/ActivityExtension/v2\"><Watts>122</Watts></TPX></Extensions></Trackpoint><Trackpoint><Time>2008-03-03T13:54:31Z</Time><Position><LatitudeDegrees>35.874856</LatitudeDegrees><LongitudeDegrees>-78.935978</LongitudeDegrees></Position><AltitudeMeters>93.866</AltitudeMeters><DistanceMeters>3389.003</DistanceMeters><Cadence>79</Cadence><Extensions><TPX xmlns=\"http://www.garmin.com/xmlschemas/ActivityExtension/v2\"><Watts>122</Watts></TPX></Extensions></Trackpoint><Trackpoint><Time>2008-03-03T13:54:32Z</Time><Position><LatitudeDegrees>35.874858</LatitudeDegrees><LongitudeDegrees>-78.935904</LongitudeDegrees></Position><AltitudeMeters>93.385</AltitudeMeters><DistanceMeters>3395.711</DistanceMeters><Cadence>79</Cadence><Extensions><TPX xmlns=\"http://www.garmin.com/xmlschemas/ActivityExtension/v2\"><Watts>116</Watts></TPX></Extensions></Trackpoint><Trackpoint><Time>2008-03-03T13:54:33Z</Time><Position><LatitudeDegrees>35.874855</LatitudeDegrees><LongitudeDegrees>-78.935829</LongitudeDegrees></Position><AltitudeMeters>93.385</AltitudeMeters><DistanceMeters>3402.468</DistanceMeters><Cadence>72</Cadence><Extensions><TPX xmlns=\"http://www.garmin.com/xmlschemas/ActivityExtension/v2\"><Watts>116</Watts></TPX></Extensions></Trackpoint><Trackpoint><Time>2008-03-03T13:54:34Z</Time><Position><LatitudeDegrees>35.874860</LatitudeDegrees><LongitudeDegrees>-78.935751</LongitudeDegrees></Position><AltitudeMeters>93.385</AltitudeMeters><DistanceMeters>3409.595</DistanceMeters><Cadence>74</Cadence><Extensions><TPX xmlns=\"http://www.garmin.com/xmlschemas/ActivityExtension/v2\"><Watts>116</Watts></TPX></Extensions></Trackpoint><Trackpoint><Time>2008-03-03T13:54:35Z</Time><Position><LatitudeDegrees>35.874870</LatitudeDegrees><LongitudeDegrees>-78.935669</LongitudeDegrees></Position><AltitudeMeters>93.385</AltitudeMeters><DistanceMeters>3417.049</DistanceMeters><Cadence>76</Cadence><Extensions><TPX xmlns=\"http://www.garmin.com/xmlschemas/ActivityExtension/v2\"><Watts>116</Watts></TPX></Extensions></Trackpoint><Trackpoint><Time>2008-03-03T13:54:36Z</Time><Position><LatitudeDegrees>35.874879</LatitudeDegrees><LongitudeDegrees>-78.935589</LongitudeDegrees></Position><AltitudeMeters>93.385</AltitudeMeters><DistanceMeters>3424.355</DistanceMeters><Cadence>76</Cadence><Extensions><TPX xmlns=\"http://www.garmin.com/xmlschemas/ActivityExtension/v2\"><Watts>115</Watts></TPX></Extensions></Trackpoint><Trackpoint><Time>2008-03-03T13:54:37Z</Time><Position><LatitudeDegrees>35.874894</LatitudeDegrees><LongitudeDegrees>-78.935507</LongitudeDegrees></Position><AltitudeMeters>93.385</AltitudeMeters><DistanceMeters>3431.981</DistanceMeters><Cadence>78</Cadence><Extensions><TPX xmlns=\"http://www.garmin.com/xmlschemas/ActivityExtension/v2\"><Watts>106</Watts></TPX></Extensions></Trackpoint><Trackpoint><Time>2008-03-03T13:54:38Z</Time><Position><LatitudeDegrees>35.874909</LatitudeDegrees><LongitudeDegrees>-78.935423</LongitudeDegrees></Position><AltitudeMeters>93.385</AltitudeMeters><DistanceMeters>3439.728</DistanceMeters><Cadence>78</Cadence><Extensions><TPX xmlns
